vi "User Input.vi"() -> ()   [LabVIEW 2013]
uses:
  <vilib>/LabVIEW Hacker/XBMC/Private/Type Defs/Input.Action.ctl
  <vilib>/LabVIEW Hacker/XBMC/LVH-XBMC.lvlib
panel:
  in  "Input Action":T1
  in  "Stop Button":bool
  out "Error Out":errorcluster
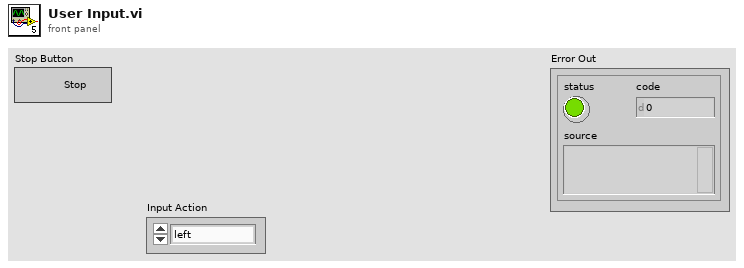
[diagram p1: front panel]
types:
  T1 = typedef "LVH-XBMC.lvlib/Input.Action.ctl" = enum16{"left", "right", "up", "down", "pageup", "pagedown", "select", "highlight", "parentdir", "parentfolder", "back", "previousmenu", "info", "pause", "stop", "skipnext", "skipprevious", "fullscreen", "aspectratio", "stepforward", "stepback", "bigstepforward", "bigstepback", "chapterorbigstepforward", "chapterorbigstepback", "osd", "showsubtitles", "nextsubtitle", "codecinfo", "nextpicture", "previouspicture", "zoomout", "zoomin", "playlist", "queue", "zoomnormal", "zoomlevel1", "zoomlevel2", "zoomlevel3", "zoomlevel4", "zoomlevel5", "zoomlevel6", "zoomlevel7", "zoomlevel8", "zoomlevel9", "nextcalibration", "resetcalibration", "analogmove", "rotate", "rotateccw", "close", "subtitledelayminus", "subtitledelay", "subtitledelayplus", "audiodelayminus", "audiodelay", "audiodelayplus", "subtitleshiftup", "subtitleshiftdown", "subtitlealign", "audionextlanguage", "verticalshiftup", "verticalshiftdown", "nextresolution", "audiotoggledigital", "number0", "number1", "number2", "number3", "number4", "number5", "number6", "number7", "number8", "number9", "osdleft", "osdright", "osdup", "osddown", "osdselect", "osdvalueplus", "osdvalueminus", "smallstepback", "fastforward", "rewind", "play", "playpause", "switchplayer", "delete", "copy", "move", "mplayerosd", "hidesubmenu", "screenshot", "rename", "togglewatched", "scanitem", "reloadkeymaps", "volumeup", "volumedown", "mute", "backspace", "scrollup", "scrolldown", "analogfastforward", "analogrewind", "moveitemup", "moveitemdown", "contextmenu", "shift", "symbols", "cursorleft", "cursorright", "showtime", "analogseekforward", "analogseekback", "showpreset", "presetlist", "nextpreset", "previouspreset", "lockpreset", "randompreset", "increasevisrating", "decreasevisrating", "showvideomenu", "enter", "increaserating", "decreaserating", "togglefullscreen", "nextscene", "previousscene", "nextletter", "prevletter", "jumpsms2", "jumpsms3", "jumpsms4", "jumpsms5", "jumpsms6", "jumpsms7", "jumpsms8", "jumpsms9", "filter", "filterclear", "filtersms2", "filtersms3", "filtersms4", "filtersms5", "filtersms6", "filtersms7", "filtersms8", "filtersms9", "firstpage", "lastpage", "guiprofile", "red", "green", "yellow", "blue", "increasepar", "decreasepar", "volampup", "volampdown", "createbookmark", "createepisodebookmark", "settingsreset", "settingslevelchange", "stereomode", "nextstereomode", "previousstereomode", "togglestereomode", "stereomodetomono", "channelup", "channeldown", "previouschannelgroup", "nextchannelgroup", "playpvr", "playpvrtv", "playpvrradio", "record", "leftclick", "rightclick", "middleclick", "doubleclick", "wheelup", "wheeldown", "mousedrag", "mousemove", "tap", "longpress", "pangesture", "zoomgesture", "rotategesture", "swipeleft", "swiperight", "swipeup", "swipedown", "noop"}
  T2 = typedef "LVH-XBMC.lvlib/XBMC Ref.ctl" = cluster{"HTTP Handle":T3, "Hostname / IP":string}
  T3 = typedef "LabVIEWHTTPClient.lvlib/ClientHandle.ctl" = refnum<k1>
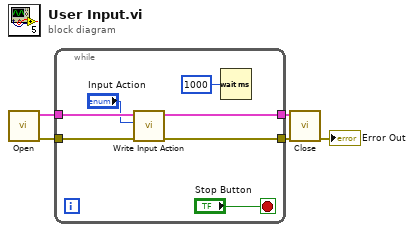
[diagram p0: block diagram]
diagram:
  n1 = call <vilib>:"Open.vi"() -> ("Error Out"=w4:errorcluster, "XBMC Ref"=w5:T2)  [unwired: 10 in]
  n2 = while {
    tunnel: w5 -> [w12]
    tunnel: w4 -> [w11]
    tunnel: [w10] -> w3
    tunnel: [w9] -> w2
    stop <- "Stop Button" stop-if-true
    n3 = call <vilib>:"Write Input Action.vi"("Error In"=w11, "Input Action"="Input Action", "XBMC Ref"=w12) -> ("Error Out"=w10:errorcluster, "XBMC Ref"=w9:T2)  [unwired: 7 in]
    n4 = Wait (ms)(milliseconds to wait=u32 1000) -> ()  [unwired: 1 out]
  }
  n5 = call <vilib>:"Close.vi"("Error In"=w3, "XBMC Ref"=w2) -> ("Error Out"=→"Error Out":errorcluster)  [unwired: 9 in]
